vi "Test Load Instruments 3.vi"(11 "Test Case In":refnum<class "Test Instrument Manager.lvclass">) -> (0 "error out":errorcluster, 3 "Test Case Out":refnum<class "Test Instrument Manager.lvclass">)   [LabVIEW 2024, in "Test Instrument Manager.lvclass"]
uses:
  Test Instrument Manager.lvclass
  C:/Program Files/National Instruments/LabVIEW 2025/vi.lib/Astemes/LUnit/Test Case.lvclass
  Alarming Strategy/Alarming Strategy.lvclass
  D:/git/HAL/Source/Interfaces/IConfigure/IConfigure.lvclass
  <vilib>/Astemes/LUnit/Test Case.lvclass/Test Case.ctl
  Test Instrument Manager.lvclass/Test Instrument Manager.ctl
  Instrument Manager/Instrument Manager.lvclass
  <vilib>/Astemes/LUnit/Test Case.lvclass
  D:/git/HAL/Source/Interfaces/IClose/IClose.lvclass
  D:/git/HAL/Source/Interfaces/IInitialize/IInitialize.lvclass
  D:/git/HAL/Source/Alarming Strategy/Alarming Strategy.lvclass
  D:/git/HAL/Source/Interfaces/ICreate Action Point/ICreate Action Point.lvclass
  C:/Program Files/National Instruments/LabVIEW 2025/vi.lib/Astemes/LUnit/LUnit Runnable.lvclass
  D:/git/HAL/Source/Tests/Test Instrument Manager/Test Instrument Manager.lvclass
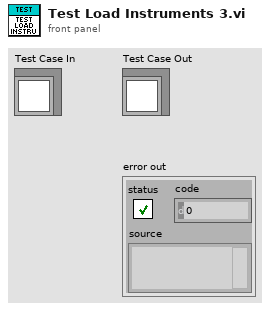
[diagram p1: front panel]
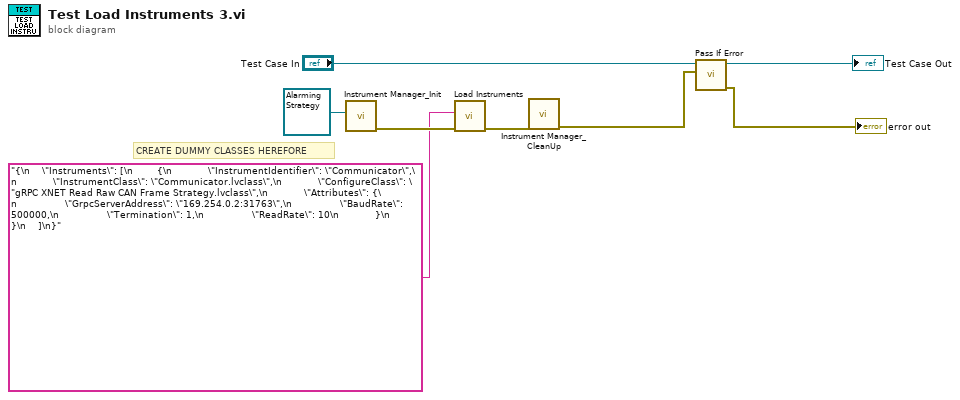
[diagram p0: block diagram]
diagram:
  # "CREATE DUMMY CLASSES HEREFORE"
  n1 = call "Instrument Manager_Init.vi"("IConfigure"=refnum<class "Alarming Strategy.lvclass"> refnum ("Alarming Strategy.lvclass")) -> ("Error Out"=w6:errorcluster)  [unwired: 9 in, 1 out]
  n2 = call "Load Instruments.vi"("Error In"=w6, "Source"="{\n    \"Instruments\": [\n        {\n            \"InstrumentIdentifier\": \"Communicator\",\n            \"InstrumentClass\": \"Communicator.lvclass\",\n            \"ConfigureClass\": \"gRPC XNET Read Raw CAN Frame Strategy.lvclass\",\n            \"Attributes\": {\n                \"GrpcServerAddress\": \"169.254.0.2:31763\",\n                \"BaudRate\": 500000,\n                \"Termination\": 1,\n                \"ReadRate\": 10\n            }\n        }\n    ]\n}") -> ("Error Out"=w5:errorcluster)  [unwired: 9 in]
  n3 = call "Instrument Manager_CleanUp.vi"("Error In"=w5) -> ("Error Out"=w4:errorcluster)  [unwired: 10 in]
  n4 = call <vilib>:"Pass If Error.vi"("Assert error"=w4, "LUnit Test Case In"="Test Case In") -> ("error out"=→"error out":errorcluster, "LUnit Test Case Out"=→"Test Case Out":refnum<class "Test Instrument Manager.lvclass">)  [unwired: 8 in]
